vi "old FGGA_10Hz_test.vi"(0 "VISA resource name out":refnum<visa-resource-name>, 11 "error IO":errorcluster) -> ()   [LabVIEW 2014]
uses:
  <vilib>/Instr/_visa.llb/VISA Set IO Buffer Mask.ctl
  <vilib>/Instr/_visa.llb/VISA Flush IO Buffer Mask.ctl
  <vilib>/Instr/_visa.llb/VISA Configure Serial Port (Instr).vi
  <vilib>/platform/TimedLoop/XDataNode/XDataNode.xnode
  <vilib>/Platform/TimedLoop/XDataNode/nitl_modes.ctl
  <vilib>/Platform/TimedLoop/XDataNode/XDNodeRunTimeDep.lvlib
  <vilib>/Platform/TimedLoop/XDataNode/wakeup.ctl
  <vilib>/Platform/TimedLoop/XDataNode/timing_clust.ctl
panel:
  out "Waveform Chart 3":u32(graph)
  out "Max time diff":u32
  out "Max time diff":u32
  out "time diff":u32(graph)
  out "Loop count 2":i32
  out "Number of times \nRead time out 2":u32
  out "RAW DATA 2":string
  out "length 2":i32
  out "Waveform Chart 2":i32(graph)
  out "Waveform Chart":i32(graph)
  out "length":i32
  out "Serial error out":errorcluster
  out "RAW DATA":string
  in  "stop":bool
  out "Number of times \nRead time out":u32
  out "Loop count":i32
  # "Date"
  # "Time"
  # "CH4_wet_ppm"
  # "1"
  # "CO4_wet_ppm_sd"
  # "H2O_ppm"
  # "3"
  # "H2O_ppm_sd"
  # "CO2_wet_ppm"
  # "5"
  # "CO2_wet_ppm_sd"
  # "CH4_dry_ppm"
  # "CH4_dry_ppm_sd"
  # "CO2_dry_ppm"
  # "CO2_dry_ppm_sd"
  # "cell_pressure_torr"
  # "11"
  # "cell_pressure_torr_sd"
  # "13"
  # "cell_temp_degC"
  # "cell_temp_degC_sdev"
  # "ambient(bench)_temp_degC"
  # "15"
  # "ambient(bench)_temp_dedgC_sd"
  # "17"
  # "RDA_us"
  # "RDA_us_sd"
  # "RDB_us"
  # "19"
  # "RDB_us_sd"
  # "Fitflag"
  # "21"
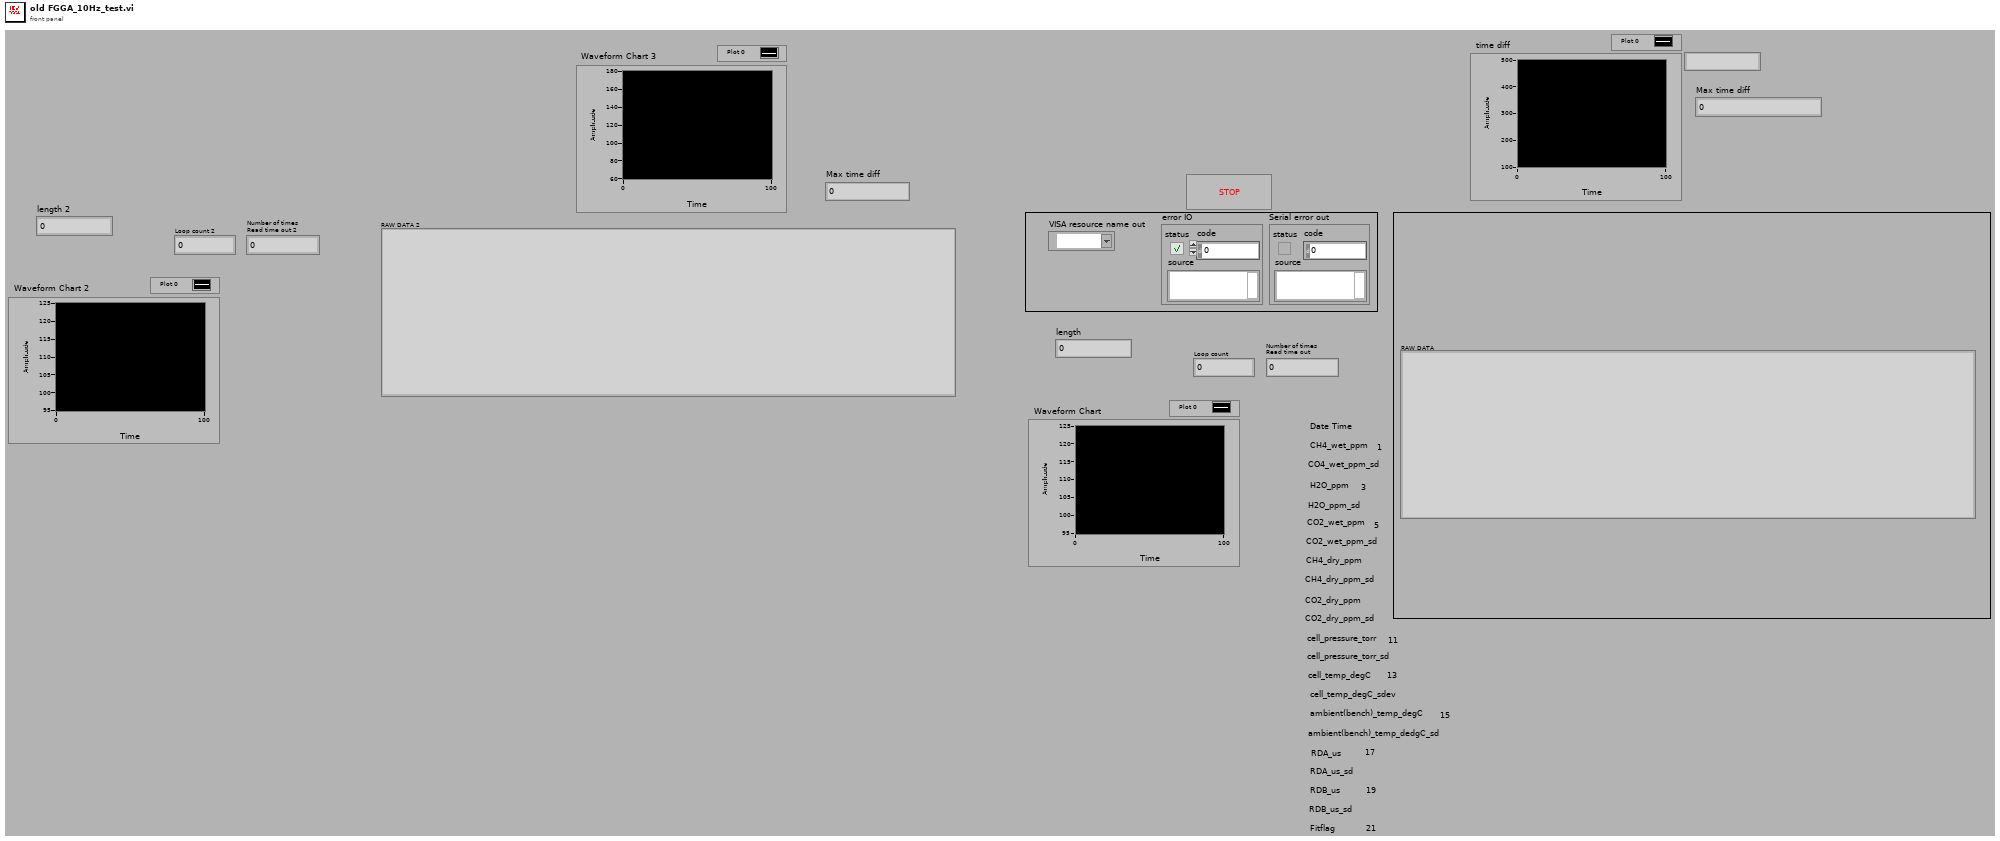
[diagram p1: front panel]
types:
  T1 = typedef "VISA Flush IO Buffer Mask.ctl" = u16
  T2 = typedef "VISA Set IO Buffer Mask.ctl" = u16
  T3 = typedef "XDNodeRunTimeDep.lvlib/timing_clust.ctl" = cluster{"Expected End [f-1]":u64, "Actual End [f-1]":u64, "Finished Late? [f-1]":bool, "Expected End [i-1]":u64, "Actual End [i-1]":u64, "Finished Late? [i-1]":bool, "Expected Start [i]":u64, "Actual Start [i]":u64, "Expected Start [f]":u64, "Actual Start [f]":u64, "Source Name":string, "Structure Name":string, "Period":i64, "Deadline":i64, "Offset":i64, "Start":i64, "Priority":i32, "Timeout":i32, "Mode":T4, "Wakeup Reason":T5, "Error":errorcluster, "Source Type":string, "Secondary Source Type":string, "Global End Time":u64, "Global Start Time":u64, "Frame Duration":u64, "Iteration Duration":u64, "Assigned CPU":i32, "I/O Scan Engine Mode":u32}
  T4 = typedef "XDNodeRunTimeDep.lvlib/nitl_modes.ctl" = enum32{"No Change", "Process missed periods, maintain original phase", "Discard missed periods, maintain original phase", "Process missed periods, ignore original phase", "Discard missed periods, ignore original phase"}
  T5 = typedef "XDNodeRunTimeDep.lvlib/wakeup.ctl" = enum32{"Normal", "Aborted", "Asynchronous wakeup", "Timing source error", "Timed loop error", "Timeout"}
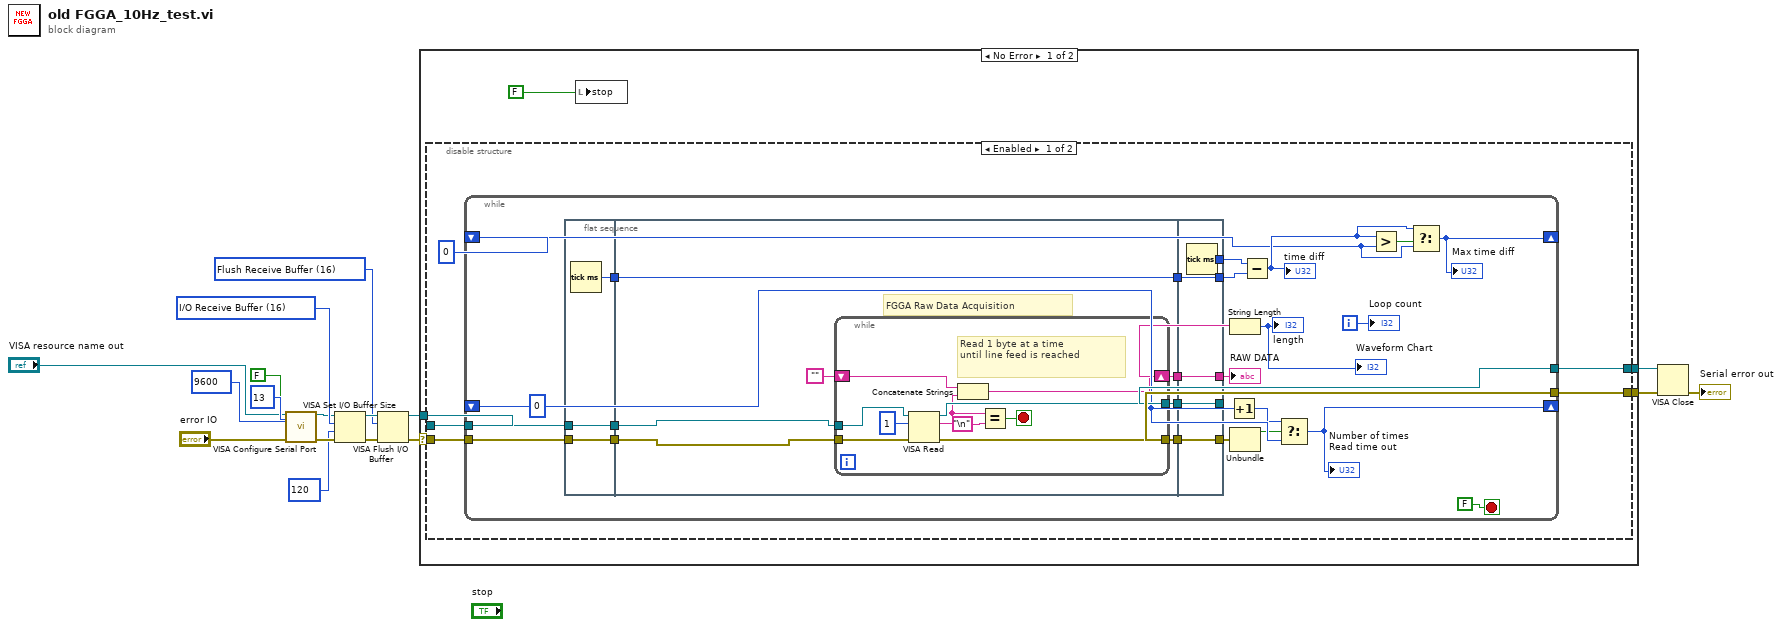
[diagram p0: block diagram]
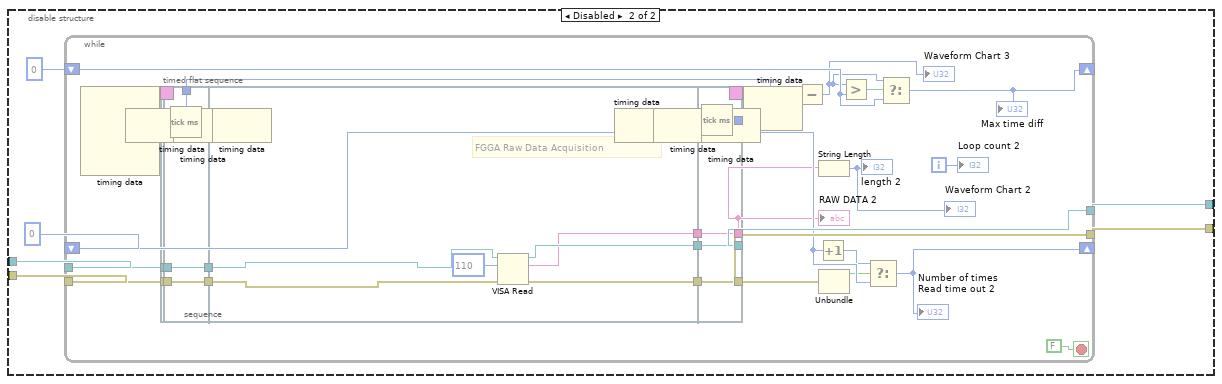
[diagram p2: hidden frame]
diagram:
  w9 = T1 16 items=["Flush Receive Buffer"=16, "Write Transmit Buffer to Device"=32, "Flush Receive Buffer (No I/O)"=64, "Flush Transmit Buffer"=128] ("Mask")
  w10 = T2 16 items=["I/O Receive Buffer"=16, "I/O Transmit Buffer"=32, "I/O Receive and Transmit Buffer"=48] ("Mask")
  n1 = call-poly "VISA Configure Serial Port"("VISA resource name"="VISA resource name out", "termination char\n(0xA = '\\n' = LF)"=u8 13 ("termination char\n(0xA = '\\n' = LF)"), "Enable Termination\nChar (T)"=FALSE ("Enable Termination\nChar (T)"), "baud rate (9600)"=u32 9600, "error in (no error)"="error IO") -> ("VISA resource name out"=w8:refnum<visa-resource-name>, "error out"=w7:errorcluster)  [unwired: 9 in]
  n2 = VISA Set I/O Buffer Size(VISA resource name=w8, mask (16)=w10, size (4096)=u32 120, error in (no error)=w7) -> (VISA resource name out=w11:refnum<visa-resource-name>, error out=w12:errorcluster)
  n3 = VISA Flush I/O Buffer(VISA resource name=w11, mask (16)=w9, error in (no error)=w12) -> (VISA resource name out=w4:refnum<visa-resource-name>, error out=w3:errorcluster)
  n4 = case shown="No Error" w3 {
    selector: w3 -> [w18 w138]
    tunnel: w4 -> [w19 w139]
    tunnel: [w21 w139] -> w15
    tunnel: [w22 w138] -> w16
    frame No Error {
      n5 = disable-structure shown="Enabled" {
        disable-tunnel: [w28 w83] -> w22
        disable-tunnel: [w27 w84] -> w21
        disable-tunnel: w19 -> [w26 w82]
        disable-tunnel: w18 -> [w25 w81]
        frame Enabled {
          n6 = while {
            tunnel: w26 -> [w43]
            tunnel: w25 -> [w42]
            tunnel: [w53] -> w28
            shift-right: [w49] -> _
            shift-left: u32 0 -> [w50]
            tunnel: [w52] -> w27
            shift-right: [w36] -> _
            shift-left: u32 0 -> [w37]
            i -> [w51]
            stop <- FALSE stop-if-true
            n7 = flat-sequence {
              tunnel: w42 -> [w55]
              tunnel: w43 -> [w56]
              tunnel: [w56] -> w30
              tunnel: [w55] -> w31
              tunnel: [w54] -> w29
              tunnel: w30 -> [w58]
              tunnel: w31 -> [w57]
              tunnel: [w63] -> w32
              tunnel: [w62] -> w33
              tunnel: [w60] -> w34
              tunnel: [w59] -> w35
              tunnel: w29 -> [w59]
              tunnel: [w76] -> w45
              tunnel: [w77] -> w52
              tunnel: [w78] -> w53
              tunnel: w32 -> [w78]
              tunnel: w33 -> [w77]
              tunnel: w34 -> [w76]
              tunnel: [w75] -> w41
              tunnel: [w74] -> w40
              tunnel: w35 -> [w74]
              frame #0 {
                n8 = Tick Count (ms)() -> (millisecond timer value=w54:u32)
              }
              frame #1 {
                # "FGGA Raw Data Acquisition"
                n9 = while {
                  tunnel: [w73] -> w62
                  tunnel: [w72] -> w63
                  tunnel: w58 -> [w71]
                  tunnel: w57 -> [w70]
                  shift-right: [w68] -> w60
                  shift-left: "" -> [w69]
                  stop <- w65 stop-if-true
                  # "Read 1 byte at a time \nuntil line feed is reached"
                  n10 = VISA Read(VISA resource name=w71, byte count=u32 1, error in (no error)=w70) -> (VISA resource name out=w73:refnum<visa-resource-name>, read buffer=w67:string, error out=w72:errorcluster)  [unwired: 1 out]
                  n11 = Concatenate Strings(w69, w67) -> (w68:string)
                  n12 = Equal?(x=w67, y="\n") -> (x = y?=w65:bool)
                }
              }
              frame #2 {
                n13 = Tick Count (ms)() -> (millisecond timer value=w75:u32)
              }
            }
            n14 = Increment(x=w50) -> (x+1=w48:u32)
            n15 = String Length(string=w45) -> (length=→"length" →"Waveform Chart":i32)
            n16 = Unbundle(w53) -> ("status"=w47:bool)  [unwired: 2 out]
            n17 = Subtract(x=w41, y=w40) -> (x-y=w38:u32)
            "time diff" <- w38
            n18 = Select(t=w48, s=w47, f=w50) -> (s? t:f=w49:u32)
            "Number of times \nRead time out" <- w49
            n19 = Greater?(x=w38, y=w37) -> (0:w39:bool)
            n20 = Select(t=w38, s=w39, f=w37) -> (s? t:f=w36:u32)
            "Max time diff" <- w36
            "Loop count" <- w51
            "RAW DATA" <- w45
          }
        }
        frame Disabled {
          n21 = while {
            tunnel: w82 -> [w95]
            tunnel: w81 -> [w94]
            tunnel: [w104] -> w83
            shift-right: [w100] -> _
            shift-left: 0 -> [w101]
            tunnel: [w103] -> w84
            shift-right: [w88] -> _
            shift-left: u32 0 -> [w89]
            i -> [w102]
            stop <- FALSE stop-if-true
            n22 = node-c288() -> (w86:T3)  [unwired: 4 in]
            n23 = timed-sequence {
              timing: w86 -> [_]
              timing-out: [_] -> w85
              tunnel: w95 -> [w116]
              tunnel: w94 -> [w115]
              tunnel: [w114] -> w91
              tunnel: [w110] -> w104
              tunnel: [w108] -> w103
              tunnel: [w106] -> w93
              tunnel: [w105] -> w92
              n24 = timed-flat-sequence {
                tunnel: w115 -> [w118]
                tunnel: w116 -> [w119]
                tunnel: [w119] -> w113
                tunnel: [w118] -> w112
                tunnel: [w117] -> w114
                tunnel: [w127] -> w111
                tunnel: [w126] -> w109
                tunnel: [w124] -> w107
                tunnel: w113 -> [w123]
                tunnel: w112 -> [w122]
                tunnel: [w131] -> w106
                tunnel: [w132] -> w108
                tunnel: [w133] -> w110
                tunnel: w111 -> [w133]
                tunnel: w109 -> [w132]
                tunnel: w107 -> [w131]
                tunnel: [w130] -> w105
                frame #0 {
                  n25 = node-c288() -> ()  [unwired: 1 in, 1 out]
                  n26 = Tick Count (ms)() -> (millisecond timer value=w117:u32)
                  n27 = node-c288() -> ()  [unwired: 1 in, 1 out]
                }
                frame #1 {
                  # "FGGA Raw Data Acquisition"
                  n28 = node-c288() -> ()  [unwired: 1 in, 1 out]
                  n29 = VISA Read(VISA resource name=w123, byte count=u32 110, error in (no error)=w122) -> (VISA resource name out=w126:refnum<visa-resource-name>, read buffer=w124:string, error out=w127:errorcluster)  [unwired: 1 out]
                  n30 = node-c288() -> ()  [unwired: 1 in, 1 out]
                }
                frame #2 {
                  n31 = node-c288() -> ()  [unwired: 1 in, 1 out]
                  n32 = Tick Count (ms)() -> (millisecond timer value=w130:u32)
                  n33 = node-c288() -> ()  [unwired: 1 in, 1 out]
                }
              }
            }
            "RAW DATA 2" <- w93
            n34 = node-c288(w85) -> ()  [unwired: 1 out]
            n35 = Subtract(x=w92, y=w91) -> (x-y=w87:u32)
            "Waveform Chart 3" <- w87
            n36 = Increment(x=w101) -> (x+1=w99:i32)
            n37 = String Length(string=w93) -> (length=→"length 2" →"Waveform Chart 2":i32)
            n38 = Unbundle(w104) -> ("status"=w98:bool)  [unwired: 2 out]
            n39 = Greater?(x=w87, y=w89) -> (0:w90:bool)
            n40 = Select(t=w99, s=w98, f=w101) -> (s? t:f=w100:i32)
            "Number of times \nRead time out 2" <- w100
            n41 = Select(t=w87, s=w90, f=w89) -> (s? t:f=w88:u32)
            "Max time diff" <- w88
            "Loop count 2" <- w102
          }
        }
      }
      n42 = local write "stop"(FALSE ("stop")) -> ()
    }
    frame Error {
    }
  }
  n43 = VISA Close(VISA resource name=w15, error in (no error)=w16) -> (error out=→"Serial error out":errorcluster)
